vi "Temperature Monitor.vi"() -> ()   [LabVIEW 2014]
doc: "This VI acquires temperature values every second. This VI also takes a running average of the last five temperature measurements and displays both the raw data and the running average in the strip chart. This VI also logs the raw data to a text file."
panel:
  in  "Stop Button":bool
  out "Temperature History":cluster{dbl, "Temperature Value":dbl}(graph)
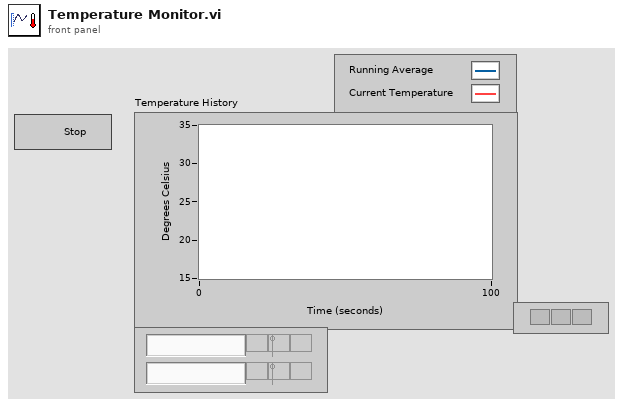
[diagram p1: front panel]
types:
  T1 = enum16{"open", "replace", "create", "open or create", "replace or create", "replace or create with confirmation"}
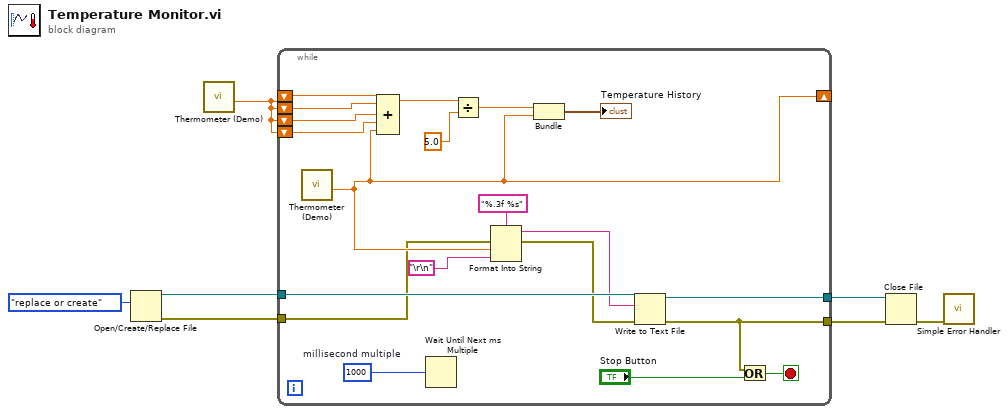
[diagram p0: block diagram]
diagram:
  n1 = Open/Create/Replace File(operation (0:open)=T1."replace or create") -> (refnum out=w2:refnum<file>, error out=w4:errorcluster)  [unwired: 1 in, 5 out]
  n2 = call "Thermometer (Demo).vi"() -> ("Temperature Value"=w7:dbl)  [unwired: 11 in]
  n3 = while {
    shift-right: [w13] -> _
    shift-left: w7 -> [w26]
    shift-left: w7 -> [w25]
    shift-left: w7 -> [w22]
    shift-left: w7 -> [w21]
    tunnel: w4 -> [w11]
    tunnel: [w16] -> w3
    tunnel: w2 -> [w18]
    tunnel: [w17] -> w1
    stop <- w14 stop-if-true
    w27 = u32 1000  # millisecond multiple
    n4 = call "Thermometer (Demo).vi"() -> ("Temperature Value"=w13:dbl)  [unwired: 11 in]
    n5 = Compound Arithmetic op=ADD(w26, w25, w22, w21, w13) -> (w24:dbl)
    n6 = Wait Until Next ms Multiple(millisecond multiple=w27) -> ()  [unwired: 1 out]
    n7 = Divide(x=w24, y=5.0) -> (x/y=w20:dbl)
    n8 = Format Into String "Format Into String"(format string="%.3f %s", error in=w11, w13, "\r\n") -> (resulting string=w12:string, error out=w10:errorcluster)  [unwired: 1 in]
    n9 = Bundle(w20, "Temperature Value"=w13) -> (→"Temperature History":cluster{dbl, "Temperature Value":dbl})  [unwired: 1 in]
    n10 = Write to Text File(file (use dialog)=w18, text=w12, error in=w10) -> (refnum out=w17:refnum<file>, error out=w16:errorcluster)  [unwired: 2 out]
    n11 = Or(x=w16, y="Stop Button") -> (x .or. y?=w14:bool)
  }
  n12 = Close File(refnum=w1, error in=w3) -> (error out=w5:errorcluster)  [unwired: 1 out]
  n13 = call <vilib>:"Simple Error Handler.vi"("error in (no error)"=w5) -> ()  [unwired: 1 in, 8 out]
